vi "Pusher_Client_IsSocketID.vi"(8 "ErrIn":errorcluster, 10 "Frame":string, 11 "Client in":refnum<class "Client.lvclass">) -> (0 "ErrOut":errorcluster, 1 "IsSocketID?":bool, 2 "socketID":string, 3 "Client out":refnum<class "Client.lvclass">)   [LabVIEW 2009, in "Client.lvclass"]
uses:
  Client.lvclass
  Client.lvclass/Client.ctl
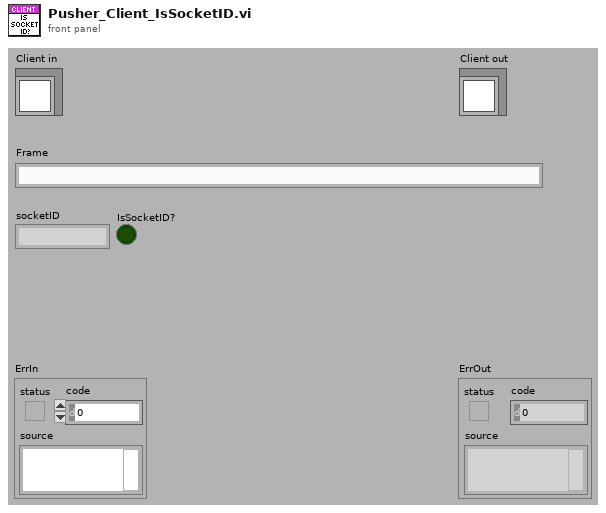
[diagram p1: front panel]
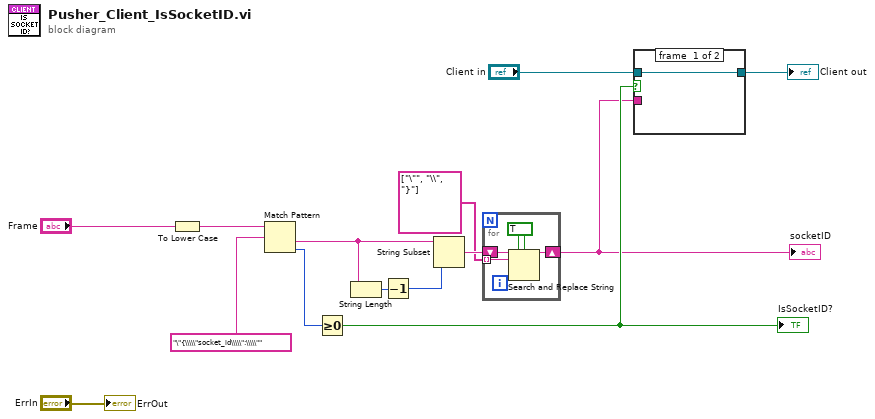
[diagram p0: block diagram]
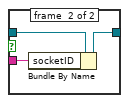
[diagram p2: hidden frame]
diagram:
  n1 = To Lower Case(string="Frame") -> (all lower case string=w4:string)
  n2 = Match Pattern(string=w4, regular expression="\"{\\\\\"socket_id\\\\\":\\\\\"") -> (after substring=w7:string, offset past match=w3:i32)  [unwired: 1 in, 2 out]
  n3 = Greater Or Equal To 0?(x=w3) -> (x >= 0?=w11:bool)
  "IsSocketID?" <- w11
  n4 = String Length(string=w7) -> (length=w6:i32)
  n5 = Decrement(x=w6) -> (x-1=w5:i32)
  n6 = String Subset(string=w7, length (rest)=w5) -> (substring=w2:string)  [unwired: 1 in]
  n7 = for {
    shift-right: [w16] -> w10
    shift-left: w2 -> [w18]
    tunnel: string[] ["\"", "\\", "}"] -> [w15] mode=indexing
    w17 = TRUE ("replace all? (F)")
    n8 = Search and Replace String(replace all?=w17, case sensitive?=w17, input string=w18, search string=w15) -> (result string=w16:string)  [unwired: 4 in, 3 out]
  }
  "socketID" <- w10
  n9 = case shown="True" w11 {
    tunnel: "Client in" -> [w19 w22]
    tunnel: [w19 w21] -> w13
    tunnel: w10 -> [_ w20]
    frame #0 {
    }
    frame #1 {
      n10 = Bundle By Name(cluster=w22, "socketID"=w20) -> (w21:refnum<class "Client.lvclass">)
    }
  }
  "Client out" <- w13
  "ErrOut" <- "ErrIn"
